vi "Example Output.vi"() -> ()   [LabVIEW 2012, in "Copy of LightPipes.lvlib"]
uses:
  Copy of LightPipes.lvlib
panel:
  out "Output":string
  in  "stop":bool
  in  "Pipe buffer size":u32=30 min=4
  in  "STD IN/OUT":u32(ring)=4294967284 items=["STD_OUTPUT_HANDLE"=4294967285, "STD_ERROR_HANDLE"=4294967284]
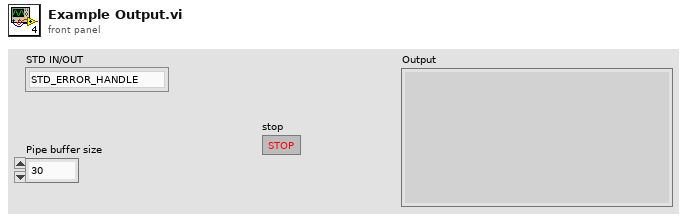
[diagram p1: front panel]
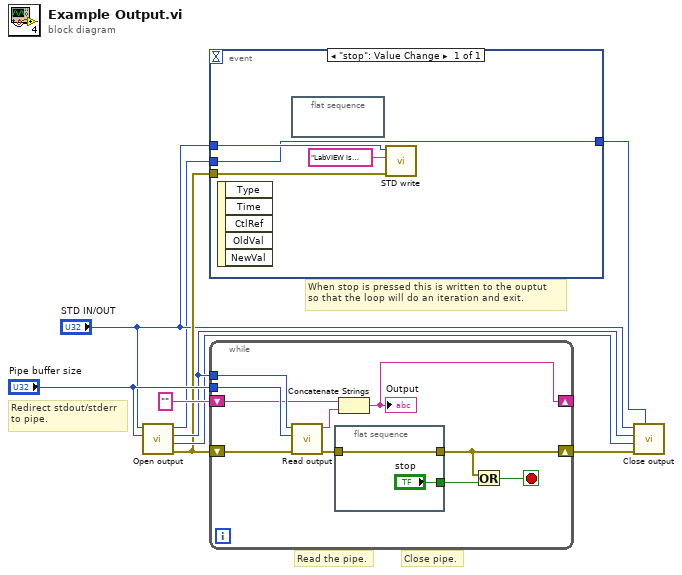
[diagram p0: block diagram]
diagram:
  # "When stop is pressed this is written to the ouptut\nso that the loop will do an iteration and exit."
  # "Close pipe."
  # "Read the pipe."
  # "Redirect stdout/stderr\nto pipe."
  n1 = call "Open output.vi"("Pipe buffer size"="Pipe buffer size", "STD IN/OUT"="STD IN/OUT") -> ("error out"=w4:errorcluster, "Write handle"=w5:u64, "Read handle"=w6:u64, "Original handle"=w2:u64)  [unwired: 6 in]
  n2 = event shown="[0] \"stop\": Value Change" {
    selector: _ -> [_]
    dyn-events: _ -> [_]
    timeout: _ -> [_]
    tunnel: w4 -> [w13]
    tunnel: "STD IN/OUT" -> [w12]
    tunnel: w2 -> [w10]
    tunnel: [w10] -> w1
    event "stop": Value Change {
      n3 = event-data() -> ()  [unwired: 1 in, 5 out]
      n4 = flat-sequence {
        frame #0 {
        }
      }
      n5 = call "STD write.vi"("error in (no error)"=w13, "Message"="LabVIEW is closing the pipe.", "STD IN/OUT"=w12) -> ()  [unwired: 7 in, 2 out]
    }
  }
  n6 = while {
    tunnel: w6 -> [w23]
    tunnel: "Pipe buffer size" -> [w22]
    shift-right: [w14] -> w7
    shift-left: w4 -> [w21]
    shift-right: [w17] -> _
    shift-left: "" ("String out") -> [w16]
    stop <- w19 stop-if-true
    n7 = call "Read output.vi"("error in (no error)"=w21, "Bytes to read"=w22, "Read handle"=w23) -> ("error out"=w15:errorcluster, "String out"=w18:string)  [unwired: 7 in]
    n8 = flat-sequence {
      tunnel: ["stop"] -> w20
      tunnel: w15 -> [w24]
      tunnel: [w24] -> w14
      frame #0 {
      }
    }
    n9 = Concatenate Strings(w16, w18) -> (w17:string)
    "Output" <- w17
    n10 = Or(x=w14, y=w20) -> (x .or. y?=w19:bool)
  }
  n11 = call "Close output.vi"("Original handle"=w1, "error in (no error)"=w7, "Write handle"=w5, "Read handle"=w6, "STD IN/OUT"="STD IN/OUT") -> ()  [unwired: 6 in, 1 out]
